vi "Read Vehicle out of Position.vi"(11 "Car Position Simulation View Definition in":refnum<class "Car Position Simulation View Definition.lvclass">) -> (3 "Car Position Simulation View Definition out":refnum<class "Car Position Simulation View Definition.lvclass">, 4 "Vehicle out of Position":bool)   [LabVIEW 2019, in "Car Position Simulation View Definition.lvclass"]
uses:
  <vilib>/gpm_packages/@cs/Car-wash/Source/Car Position Simulation View Definition/Car Position Simulation View Definition/Car Position Simulation View Definition.lvclass
  <vilib>/gpm_packages/@cs/Car-wash/Source/Car Position Simulation View Definition/Car Position Simulation View Definition/Car Position Simulation View Definition.lvclass/Car Position Simulation View Definition.ctl
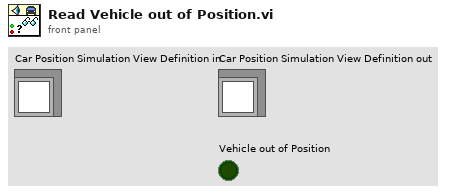
[diagram p1: front panel]
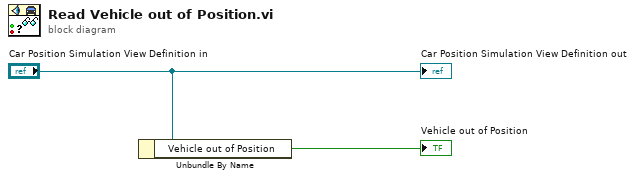
[diagram p0: block diagram]
diagram:
  n1 = Unbundle By Name("Car Position Simulation View Definition in") -> ("Vehicle out of Position"=→"Vehicle out of Position":bool)
  "Car Position Simulation View Definition out" <- "Car Position Simulation View Definition in"
